vi "Pre Launch Init.vi"(11 "Feeder in":refnum<class "Feeder.lvclass">) -> (0 "error out":errorcluster, 3 "Feeder out":refnum<class "Feeder.lvclass">)   [LabVIEW 2018, in "Feeder Actor.lvlib" / "Feeder.lvclass"]
doc: "(<B>Filename</B>: Actor Framework.lvlib:Actor.lvclass:Pre Launch Init.vi)\n\nDefines behavior that occurs after the Launch Nested Actor method is invoked but before the actor's Actor Core method begins running.\n\nBy default, this method does nothing. A descendant class may override it to define behavior."
uses:
  Feeder.lvclass
  <vilib>/ActorFramework/Actor/Actor.lvclass
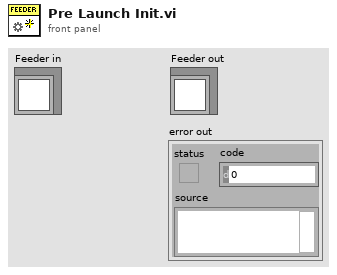
[diagram p1: front panel]
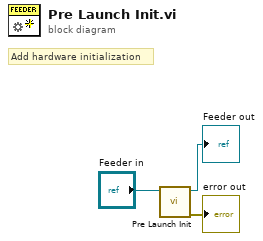
[diagram p0: block diagram]
diagram:
  # "Add hardware initialization"
  n1 = call-parent "Pre Launch Init.vi"("Actor in"="Feeder in") -> ("error out"=→"error out":errorcluster, "Actor out"=→"Feeder out":refnum<class "Feeder.lvclass">)  [unwired: 9 in]
